vi "ATF-string enable disable.vi"(8 "error in":errorcluster, 10 "Disabled":T1(ring), 11 "IP ADDRESS":refnum<vi>) -> (0 "error out":errorcluster)   [LabVIEW 2022 SP3]
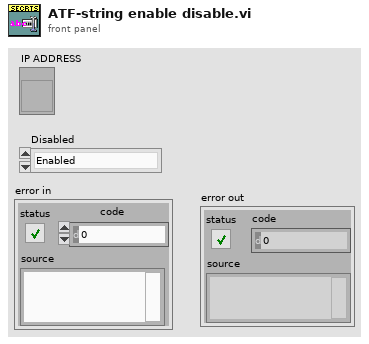
[diagram p1: front panel]
types:
  T1 = enum8{"Enabled", "Disabled", "Disabled and Grayed Out"}
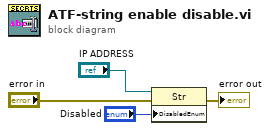
[diagram p0: block diagram]
diagram:
  n1 = property on="Property Node" class="Str"(reference="IP ADDRESS", error in="error in", "DisabledEnum"="Disabled") -> (error out=→"error out":errorcluster)  [unwired: 1 out]
